vi "IsOnConPane.vi"(6 "error in":errorcluster, 9 "Control Terminal in":refnum<class "ControlTerminal.lvclass">) -> (0 "error out":errorcluster, 2 "wired":bool, 3 "Control Terminal out":refnum<class "ControlTerminal.lvclass">, 4 "terminal index":i32)   [LabVIEW 2014, in "ControlTerminal.lvclass"]
uses:
  ControlTerminal.lvclass
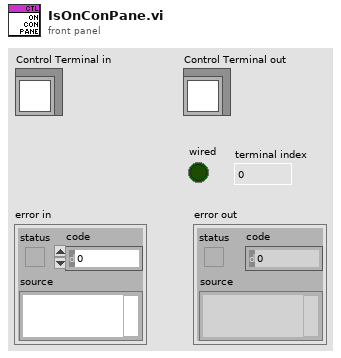
[diagram p1: front panel]
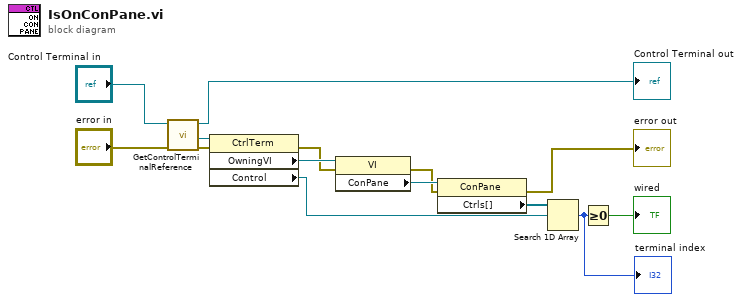
[diagram p0: block diagram]
diagram:
  n1 = call "GetControlTerminalReference.vi"("error in"="error in", "ControlTerminal in"="Control Terminal in") -> ("error out"=w6:errorcluster, "reference"=w5:refnum<vi>, "ControlTerminal out"=→"Control Terminal out":refnum<class "ControlTerminal.lvclass">)  [unwired: 7 in]
  n2 = property class="CtrlTerm"(reference=w5, error in=w6) -> (error out=w9:errorcluster, "OwningVI"=w12:refnum<vi>, "Control"=w7:refnum<vi>)  [unwired: 1 out]
  n3 = property class="VI"(reference=w12, error in=w9) -> (error out=w10:errorcluster, "ConPane"=w11:refnum<vi>)  [unwired: 1 out]
  n4 = property class="ConPane"(reference=w11, error in=w10) -> (error out=→"error out":errorcluster, "Ctrls[]"=w8:refnum<vi>[])  [unwired: 1 out]
  n5 = Search 1D Array(1D array=w8, element=w7) -> (index of element=w2:i32)  [unwired: 1 in]
  "terminal index" <- w2
  n6 = Greater Or Equal To 0?(x=w2) -> (x >= 0?=→"wired":bool)
